vi "Electrical_Potentiometer.vi"() -> ()   [LabVIEW 2020]
panel:
  in  "stop":bool
  out "?":dbl
  out "Vout":dbl
  in  "Vin":dbl(slide) scale=0.0..220.0
  out "?":dbl
  in  "Rvar":dbl(knob) scale=0.0..100.0
  in  "Rcts":dbl
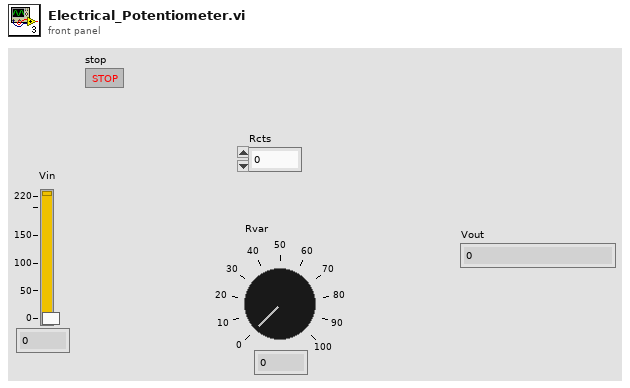
[diagram p1: front panel]
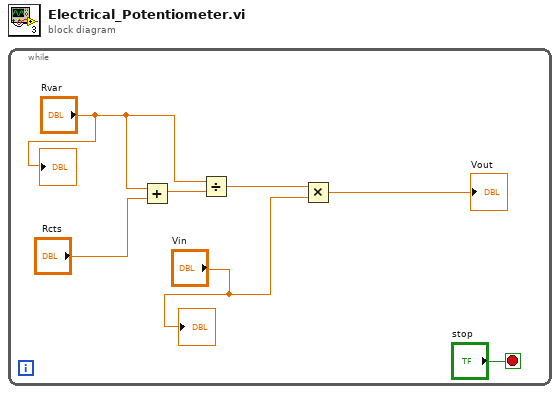
[diagram p0: block diagram]
diagram:
  n1 = while {
    stop <- "stop" stop-if-true
    n2 = Add(x="Rvar", y="Rcts") -> (x+y=w6:dbl)
    n3 = Divide(x="Rvar", y=w6) -> (x/y=w4:dbl)
    n4 = Multiply(x=w4, y="Vin") -> (x*y=→"Vout":dbl)
    "?" <- "Rvar"
    "?" <- "Vin"
  }
